vi "Message Send.vi"(8 "error in":errorcluster, 11 "EF20 in":refnum<class "EF20.lvclass">) -> (0 "error out":errorcluster, 3 "EF20 out":refnum<class "EF20.lvclass">)   [LabVIEW 2018, in "EF20.lvlib" / "EF20.lvclass"]
uses:
  EF20.lvclass
  EF20.lvclass/EF20.ctl
  PPLs/Oven/Oven.lvlibp/Oven.lvclass
  C:/Projects/LabVIEW/PPLs/Oven/Oven.lvlibp/Oven.lvclass
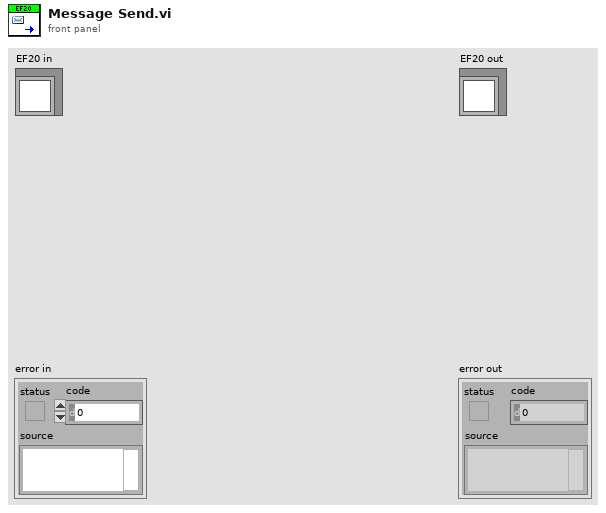
[diagram p1: front panel]
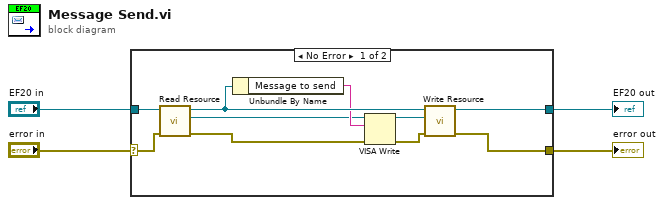
[diagram p0: block diagram]
diagram:
  n1 = case shown="No Error" "error in" {
    selector: "error in" -> [w10 w16]
    tunnel: [w9 w16] -> w3
    tunnel: [w13 w15] -> w1
    tunnel: "EF20 in" -> [w14 w15]
    frame No Error {
      n2 = call "Read Resource.vi"("error in (no error)"=w10, "Oven in"=w14) -> ("error out"=w5:errorcluster, "Resource"=w6:refnum<visa-resource-name>, "Oven out"=w8:refnum<class "EF20.lvclass">)  [unwired: 7 in]
      n3 = Unbundle By Name(w8) -> ("Message to send"=w7:string)
      n4 = VISA Write(VISA resource name=w6, write buffer=w7, error in (no error)=w5) -> (VISA resource name out=w12:refnum<visa-resource-name>, error out=w11:errorcluster)  [unwired: 1 out]
      n5 = call "Write Resource.vi"("error in (no error)"=w11, "Resource"=w12, "Oven in"=w8) -> ("error out"=w9:errorcluster, "Oven out"=w13:refnum<class "EF20.lvclass">)  [unwired: 7 in]
    }
    frame Error {
    }
  }
  "error out" <- w3
  "EF20 out" <- w1
